vi "writeLogHeader.vi"(0 "Path In":path) -> (1 "Path Out":path, 2 "refnum out":refnum<file>)   [LabVIEW 2017]
panel:
  out "concatenated string":string
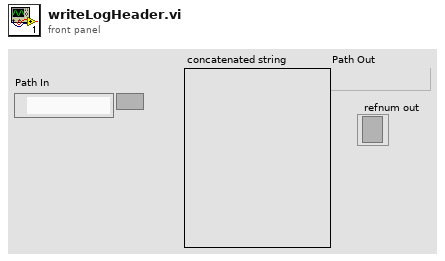
[diagram p1: front panel]
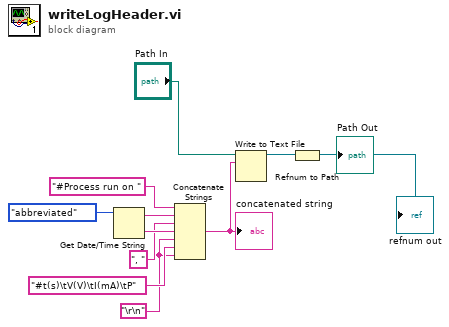
[diagram p0: block diagram]
diagram:
  w5 = "\r\n"
  n1 = Get Date/Time String(date format (0)=enum16{"short", "long", "abbreviated"}."abbreviated") -> (date string=w10:string, time string=w7:string)  [unwired: 2 in]
  n2 = Concatenate Strings("#Process run on " ("string"), w10, ", " ("string"), w7, w5, "#t(s)\tV(V)\tI(mA)\tP" ("string"), w5) -> (w9:string)
  "concatenated string" <- w9
  n3 = Write to Text File(file (use dialog)="Path In", text=w9) -> (refnum out=w3:refnum<file>)  [unwired: 2 in, 2 out]
  "refnum out" <- w3
  n4 = Refnum to Path(1:w3) -> (0:→"Path Out":path)
